vi "Motor-Maker-Triangle 2 RD.vi"() -> ()   [LabVIEW 2021]
panel:
  out "Motor Y\nLigado ida 2":bool=TRUE
  in  "stop Y descida":bool
  out "Posit Y descida":sgl
  out "Num Y descida":i32
  in  "Y descida":dbl
  out "Motor X\nLigado ida 3":bool=TRUE
  in  "stop X volta":bool
  out "Position X volta":sgl
  out "Nu X volta":i32
  in  "X volta":dbl
  out "Motor X\nLigado ida 2":bool=TRUE
  in  "stop X 2":bool
  out "pfPosition X ida 2":sgl
  out "Numeric X ida 2":i32
  in  "X ida 2":dbl
  out "Motor Y\nLigado ida":bool=TRUE
  in  "stop Y":bool
  out "Posit Y subida":sgl
  out "Num Y Subida":i32
  in  "Ysubida":dbl
  out "Motor X\nLigado ida":bool=TRUE
  in  "stop X":bool
  out "pfPosition X ida":sgl
  out "Numeric X ida":i32
  in  "X ida":dbl
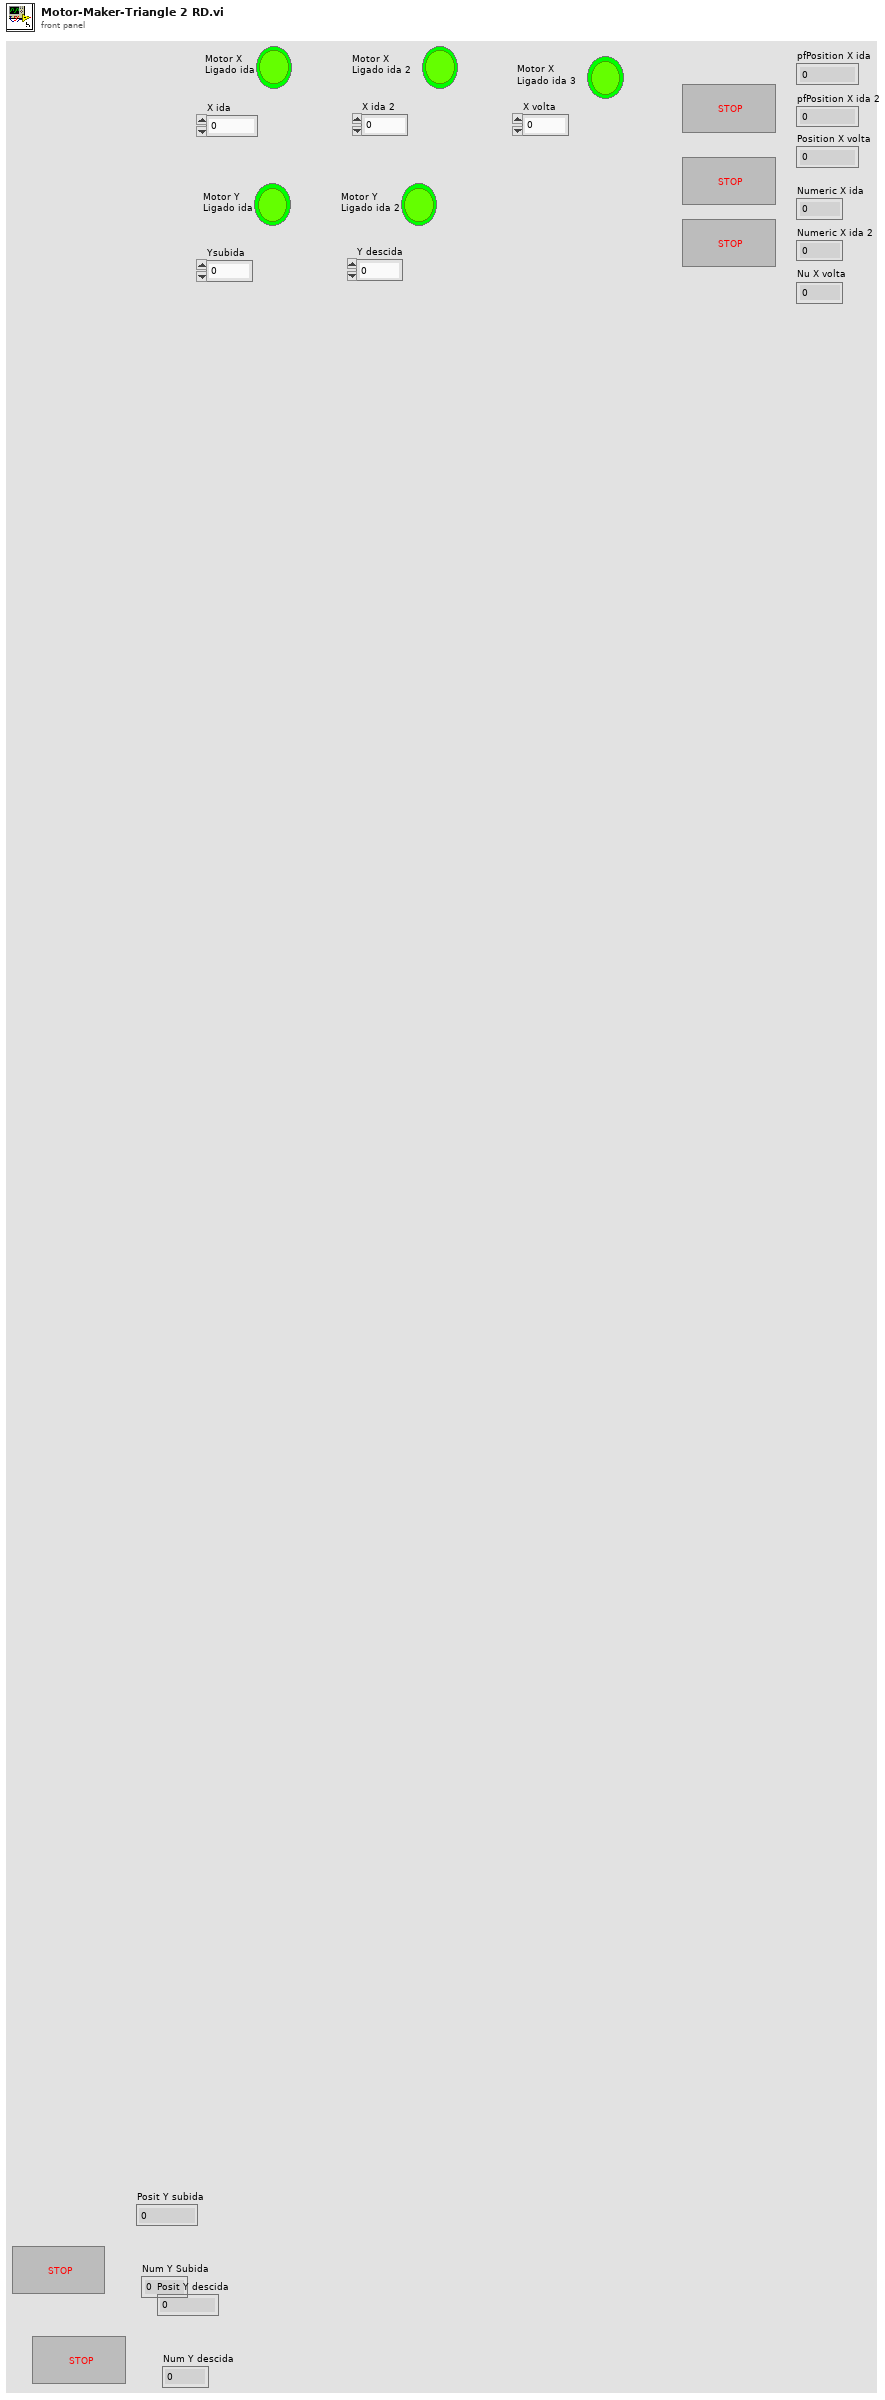
[diagram p1: front panel]
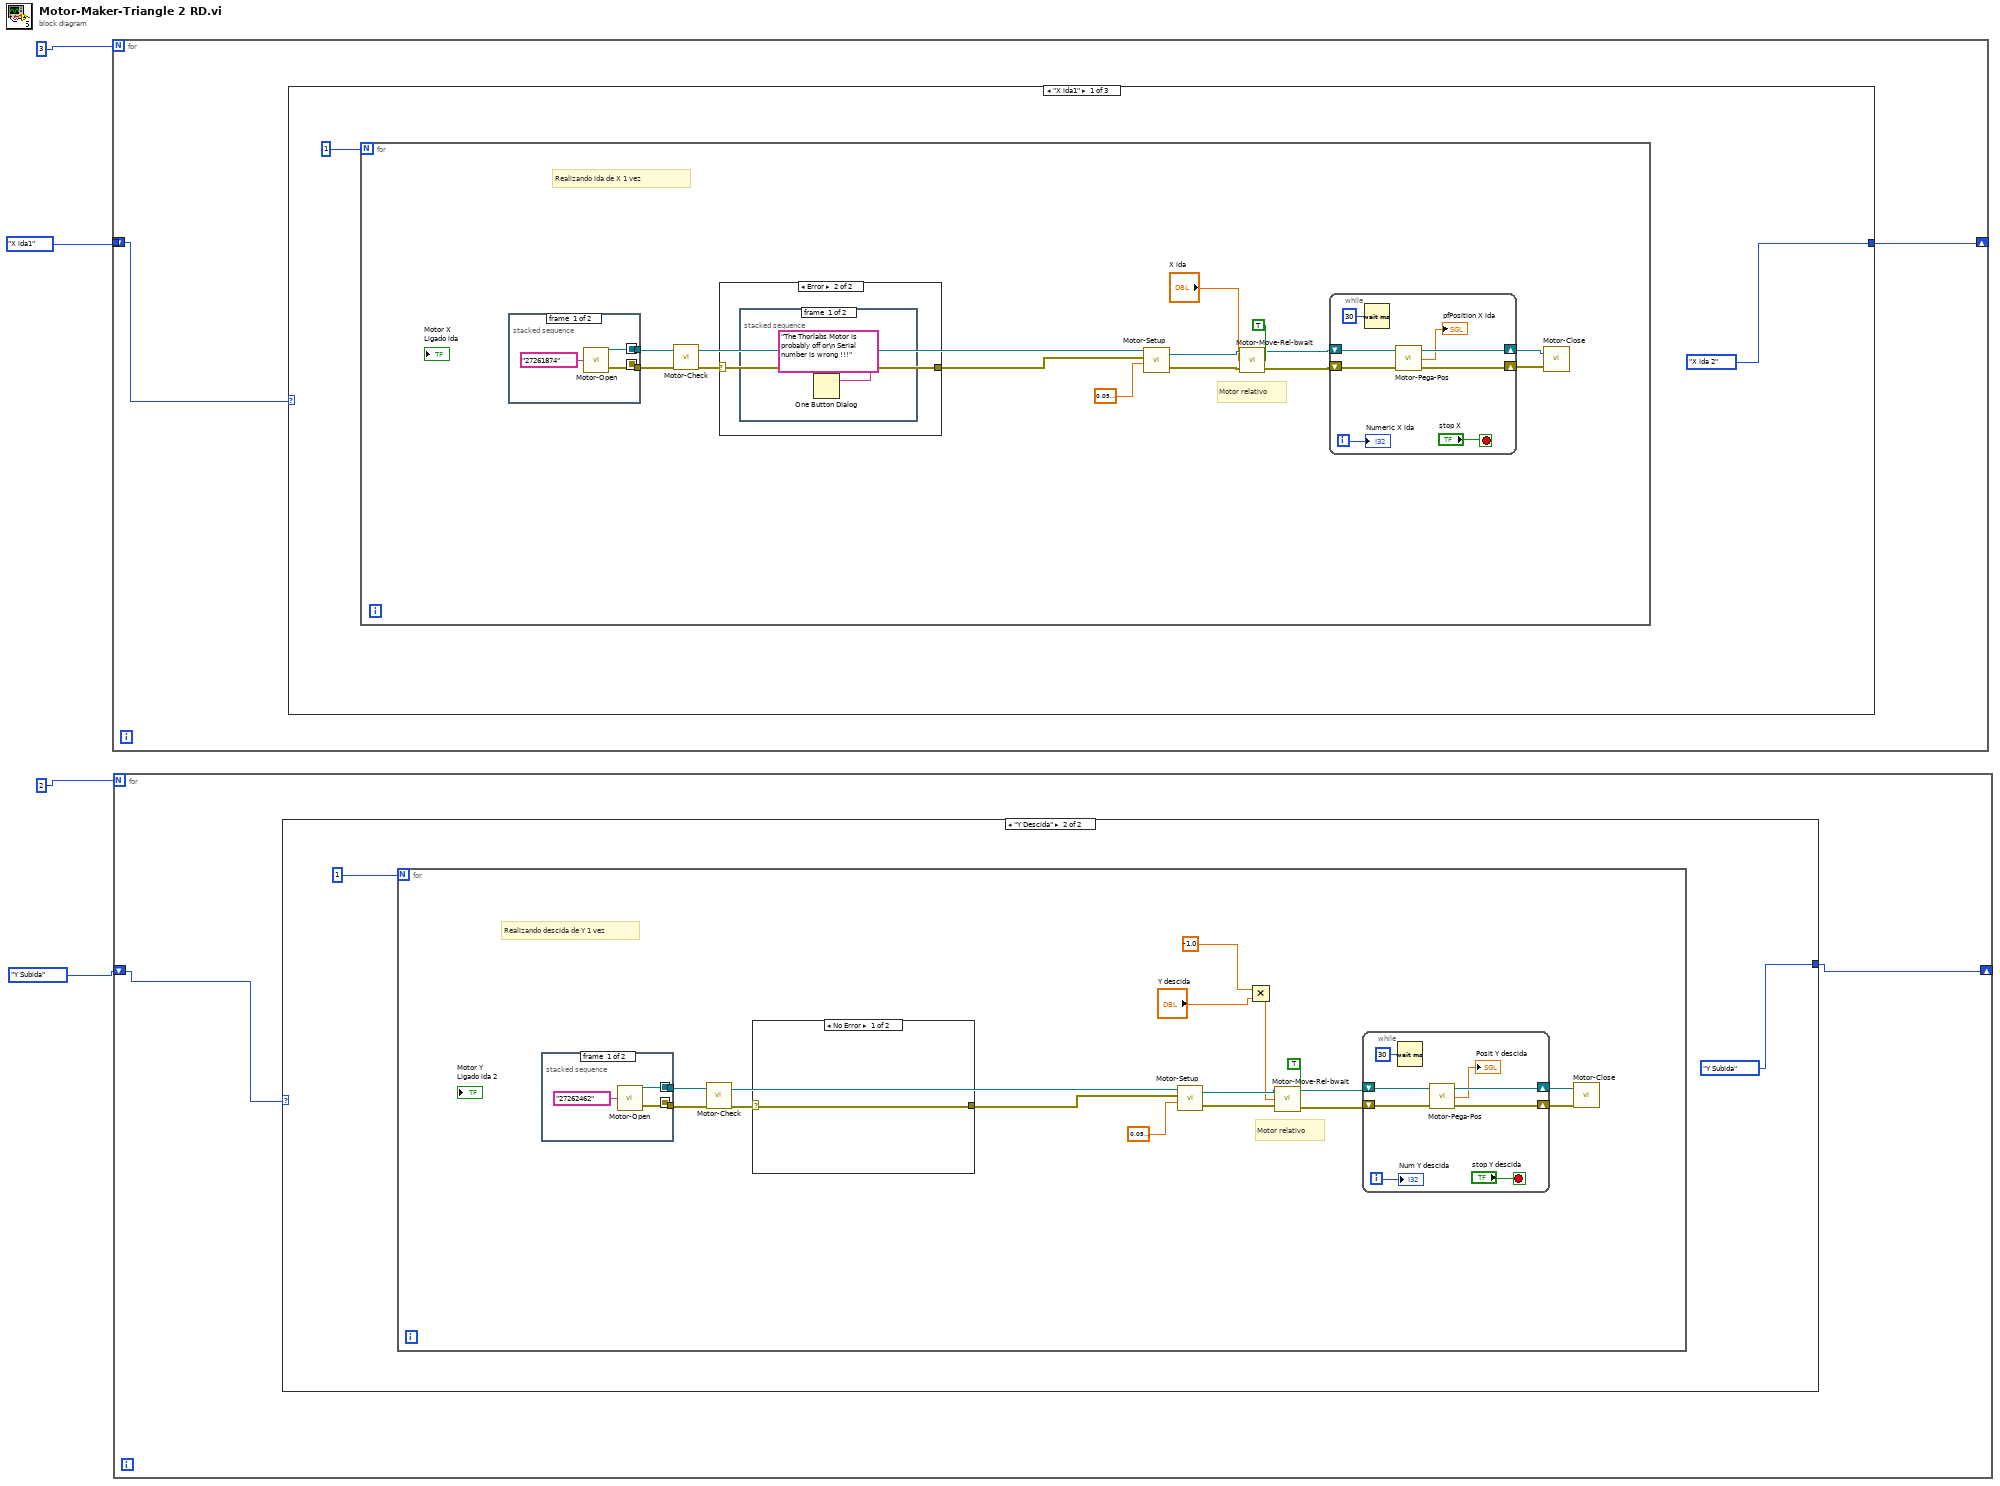
[diagram p0: block diagram]
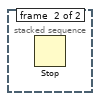
[diagram p3: hidden frame]
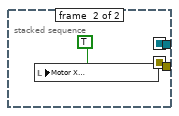
[diagram p4: hidden frame]
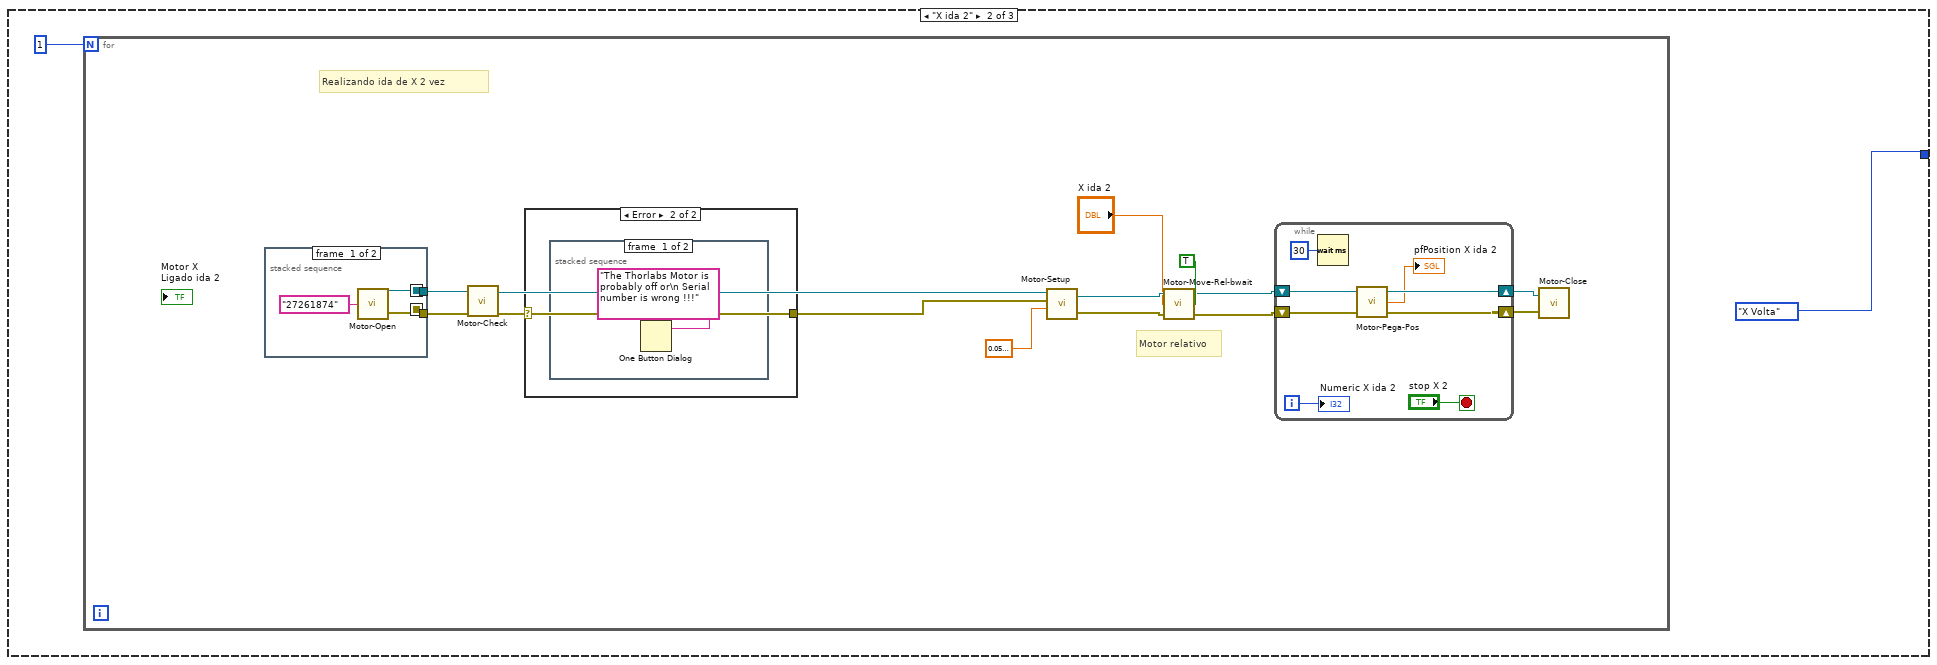
[diagram p5: hidden frame]
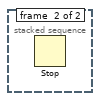
[diagram p7: hidden frame]
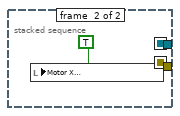
[diagram p8: hidden frame]
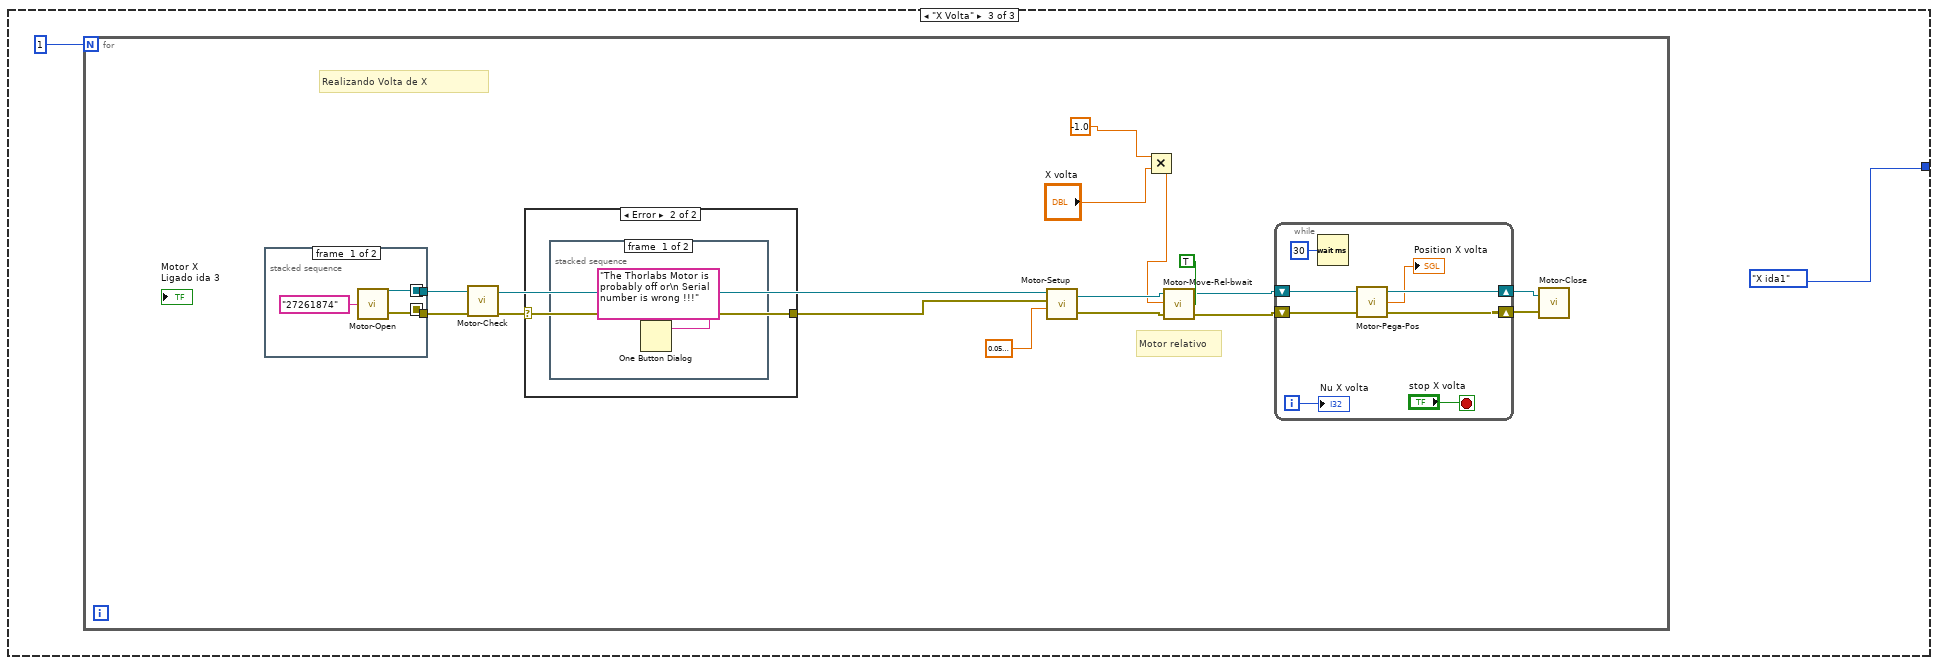
[diagram p9: hidden frame]
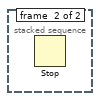
[diagram p11: hidden frame]
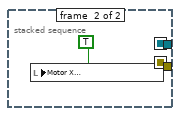
[diagram p12: hidden frame]
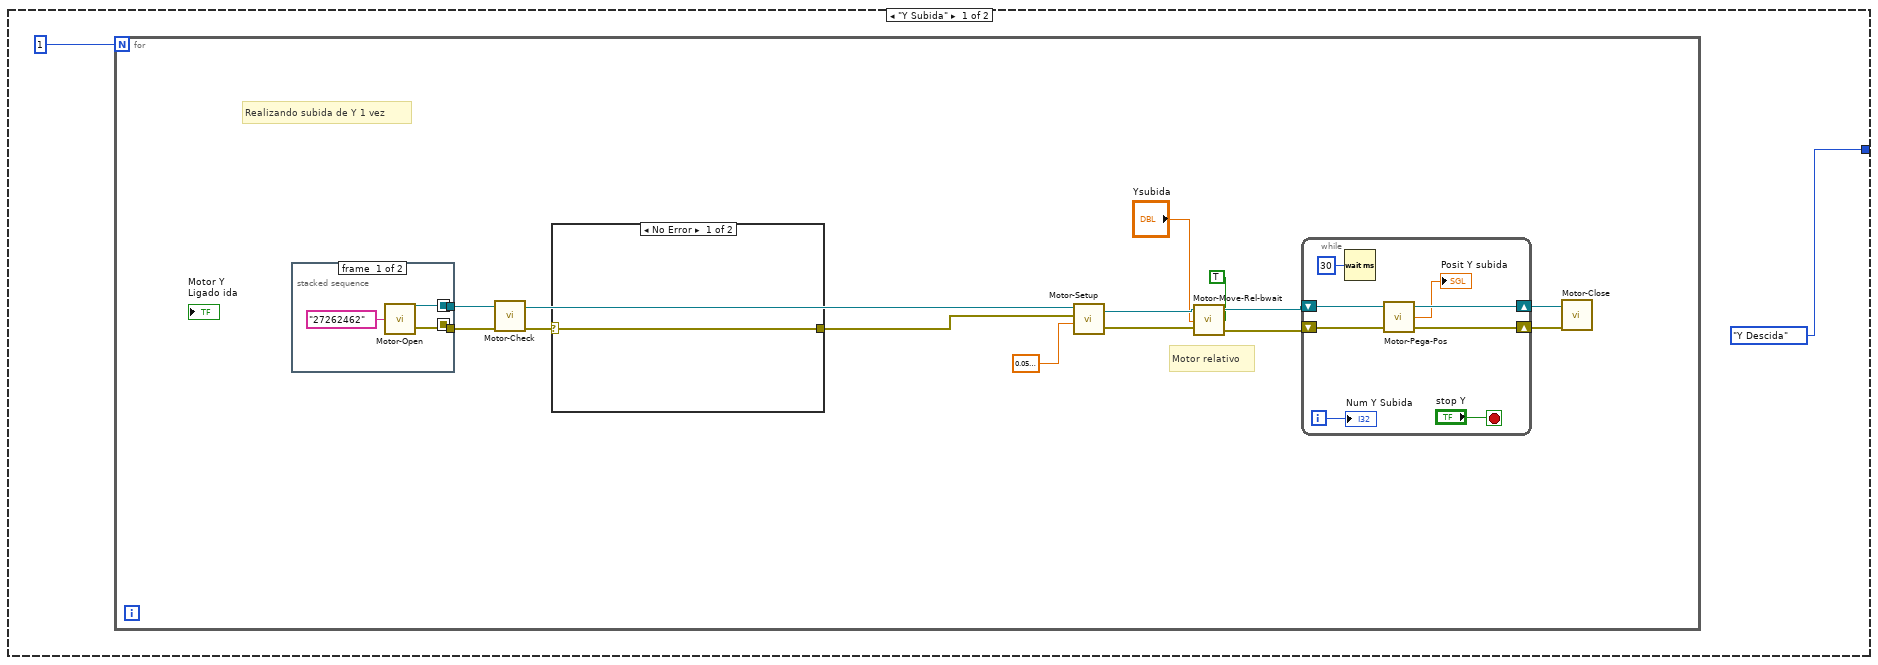
[diagram p13: hidden frame]
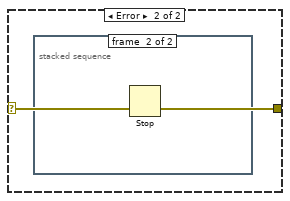
[diagram p14: hidden frame]
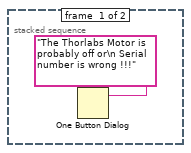
[diagram p15: hidden frame]
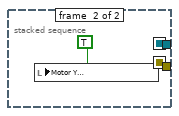
[diagram p16: hidden frame]
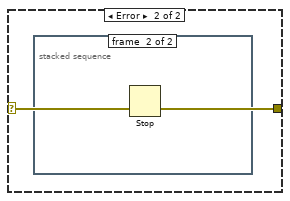
[diagram p17: hidden frame]
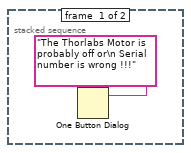
[diagram p18: hidden frame]
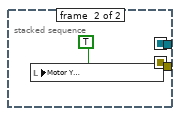
[diagram p19: hidden frame]
diagram:
  n1 = for {
    N: 3 -> [_]
    shift-right: [w6] -> _
    shift-left: _ -> [_]
    tunnel: enum16{"X ida1", "X Volta", "X ida 2"}."X ida1" -> [w5]
    n2 = case shown="\"X ida1\"" w5 {
      tunnel: [enum16{"X ida1", "X Volta", "X ida 2"}."X ida 2" enum16{"X ida1", "X Volta", "X ida 2"}."X Volta" enum16{"X ida1", "X Volta", "X ida 2"}."X ida1"] -> w6
      frame "X ida1" {
        n3 = for {
          N: 1 -> [_]
          # "Realizando ida de X 1 vez"
          # "Motor relativo"
          n4 = stacked-sequence {
            seq-local: [w36 _] -> [_ w39]
            seq-local: [w35 _] -> [_ w38]
            tunnel: [_ w39] -> w22
            tunnel: [_ w38] -> w21
            frame #0 {
              n5 = call "Motor-Open.vi"("S/N Motor"="27261874") -> ("MG17Motor 2"=w36:refnum<k7>, "error out"=w35:errorcluster)
            }
            frame #1 {
              n6 = local write "Motor X\nLigado ida"(TRUE ("Motor3\nLigado")) -> ()
            }
          }
          n7 = call "Motor-Check.vi"("error in (no error)"=w21, "Automation Refnum in"=w22) -> ("error out"=w20:errorcluster, "Automation Refnum out"=w19:refnum<k7>)  [unwired: 8 in]
          n8 = case shown="Error" w20 {
            selector: w20 -> [w23 w24]
            tunnel: [w23 w24] -> w18
            frame No Error {
            }
            frame Error {
              n9 = stacked-sequence {
                frame #0 {
                  n10 = One Button Dialog(message="The Thorlabs Motor is probably off or\n Serial number is wrong !!!") -> ()  [unwired: 1 in, 1 out]
                }
                frame #1 {
                  n11 = Stop() -> ()  [unwired: 1 in]
                }
              }
            }
          }
          n12 = call "Motor-Setup.vi"("Velocidade"=sgl 0.05, "error"=w18, "MG17Motor A"=w19) -> ("error out"=w12:errorcluster, "MG17Motor out"=w13:refnum<k7>)  [unwired: 1 in]
          n13 = call "Motor-Move-Rel-bwait.vi"("bWait"=TRUE, "error"=w12, "Posição"="X ida", "MG17Motor A"=w13) -> ("error out"=w9:errorcluster, "MG17Motor out"=w10:refnum<k7>)
          n14 = while {
            shift-right: [w31] -> w15
            shift-left: w10 -> [w33]
            shift-right: [w30] -> w16
            shift-left: w9 -> [w32]
            i -> [w26]
            stop <- "stop X" stop-if-true
            n15 = Wait (ms)(milliseconds to wait=u32 30) -> ()  [unwired: 1 out]
            n16 = call "Motor-Pega-Pos.vi"("MG17Motor 2"=w33, "error out"=w32) -> ("MG17Motor 3"=w31:refnum<k7>, "pfPosition"=→"pfPosition X ida":sgl, "error out 2"=w30:errorcluster)
            "Numeric X ida" <- w26
          }
          n17 = call "Motor-Close.vi"("error out"=w16, "MG17Motor 3"=w15) -> ()  [unwired: 1 in]
        }
      }
      frame "X ida 2" {
        n18 = for {
          N: 1 -> [_]
          # "Realizando ida de X 2 vez"
          # "Motor relativo"
          n19 = stacked-sequence {
            seq-local: [w69 _] -> [_ w72]
            seq-local: [w68 _] -> [_ w71]
            tunnel: [_ w72] -> w55
            tunnel: [_ w71] -> w54
            frame #0 {
              n20 = call "Motor-Open.vi"("S/N Motor"="27261874") -> ("MG17Motor 2"=w69:refnum<k7>, "error out"=w68:errorcluster)
            }
            frame #1 {
              n21 = local write "Motor X\nLigado ida 2"(TRUE ("Motor3\nLigado")) -> ()
            }
          }
          n22 = call "Motor-Check.vi"("error in (no error)"=w54, "Automation Refnum in"=w55) -> ("error out"=w53:errorcluster, "Automation Refnum out"=w52:refnum<k7>)  [unwired: 8 in]
          n23 = case shown="Error" w53 {
            selector: w53 -> [w56 w57]
            tunnel: [w56 w57] -> w51
            frame No Error {
            }
            frame Error {
              n24 = stacked-sequence {
                frame #0 {
                  n25 = One Button Dialog(message="The Thorlabs Motor is probably off or\n Serial number is wrong !!!") -> ()  [unwired: 1 in, 1 out]
                }
                frame #1 {
                  n26 = Stop() -> ()  [unwired: 1 in]
                }
              }
            }
          }
          n27 = call "Motor-Setup.vi"("Velocidade"=sgl 0.05, "error"=w51, "MG17Motor A"=w52) -> ("error out"=w45:errorcluster, "MG17Motor out"=w46:refnum<k7>)  [unwired: 1 in]
          n28 = call "Motor-Move-Rel-bwait.vi"("bWait"=TRUE, "error"=w45, "Posição"="X ida 2", "MG17Motor A"=w46) -> ("error out"=w42:errorcluster, "MG17Motor out"=w43:refnum<k7>)
          n29 = while {
            shift-right: [w64] -> w48
            shift-left: w43 -> [w66]
            shift-right: [w63] -> w49
            shift-left: w42 -> [w65]
            i -> [w59]
            stop <- "stop X 2" stop-if-true
            n30 = Wait (ms)(milliseconds to wait=u32 30) -> ()  [unwired: 1 out]
            n31 = call "Motor-Pega-Pos.vi"("MG17Motor 2"=w66, "error out"=w65) -> ("MG17Motor 3"=w64:refnum<k7>, "pfPosition"=→"pfPosition X ida 2":sgl, "error out 2"=w63:errorcluster)
            "Numeric X ida 2" <- w59
          }
          n32 = call "Motor-Close.vi"("error out"=w49, "MG17Motor 3"=w48) -> ()  [unwired: 1 in]
        }
      }
      frame "X Volta" {
        n33 = for {
          N: 1 -> [_]
          # "Realizando Volta de X"
          # "Motor relativo"
          n34 = stacked-sequence {
            seq-local: [w104 _] -> [_ w107]
            seq-local: [w103 _] -> [_ w106]
            tunnel: [_ w107] -> w90
            tunnel: [_ w106] -> w89
            frame #0 {
              n35 = call "Motor-Open.vi"("S/N Motor"="27261874") -> ("MG17Motor 2"=w104:refnum<k7>, "error out"=w103:errorcluster)
            }
            frame #1 {
              n36 = local write "Motor X\nLigado ida 3"(TRUE ("Motor3\nLigado")) -> ()
            }
          }
          n37 = call "Motor-Check.vi"("error in (no error)"=w89, "Automation Refnum in"=w90) -> ("error out"=w88:errorcluster, "Automation Refnum out"=w87:refnum<k7>)  [unwired: 8 in]
          n38 = case shown="Error" w88 {
            selector: w88 -> [w91 w92]
            tunnel: [w91 w92] -> w86
            frame No Error {
            }
            frame Error {
              n39 = stacked-sequence {
                frame #0 {
                  n40 = One Button Dialog(message="The Thorlabs Motor is probably off or\n Serial number is wrong !!!") -> ()  [unwired: 1 in, 1 out]
                }
                frame #1 {
                  n41 = Stop() -> ()  [unwired: 1 in]
                }
              }
            }
          }
          n42 = call "Motor-Setup.vi"("Velocidade"=sgl 0.05, "error"=w86, "MG17Motor A"=w87) -> ("error out"=w80:errorcluster, "MG17Motor out"=w81:refnum<k7>)  [unwired: 1 in]
          n43 = Multiply(x=-1.0, y="X volta") -> (x*y=w75:dbl)
          n44 = call "Motor-Move-Rel-bwait.vi"("bWait"=TRUE, "error"=w80, "Posição"=w75, "MG17Motor A"=w81) -> ("error out"=w78:errorcluster, "MG17Motor out"=w79:refnum<k7>)
          n45 = while {
            shift-right: [w99] -> w83
            shift-left: w79 -> [w101]
            shift-right: [w98] -> w84
            shift-left: w78 -> [w100]
            i -> [w94]
            stop <- "stop X volta" stop-if-true
            n46 = Wait (ms)(milliseconds to wait=u32 30) -> ()  [unwired: 1 out]
            n47 = call "Motor-Pega-Pos.vi"("MG17Motor 2"=w101, "error out"=w100) -> ("MG17Motor 3"=w99:refnum<k7>, "pfPosition"=→"Position X volta":sgl, "error out 2"=w98:errorcluster)
            "Nu X volta" <- w94
          }
          n48 = call "Motor-Close.vi"("error out"=w84, "MG17Motor 3"=w83) -> ()  [unwired: 1 in]
        }
      }
    }
  }
  n49 = for {
    N: 2 -> [_]
    shift-right: [w108] -> _
    shift-left: enum16{"Y Subida", "Y Descida"}."Y Subida" -> [w109]
    n50 = case shown="\"Y Descida\"" w109 {
      tunnel: [enum16{"Y Subida", "Y Descida"}."Y Descida" enum16{"Y Subida", "Y Descida"}."Y Subida"] -> w108
      frame "Y Subida" {
        n51 = for {
          N: 1 -> [_]
          # "Realizando subida de Y 1 vez"
          # "Motor relativo"
          n52 = stacked-sequence {
            seq-local: [w139 _] -> [_ w142]
            seq-local: [w138 _] -> [_ w141]
            tunnel: [_ w142] -> w123
            tunnel: [_ w141] -> w122
            frame #0 {
              n53 = call "Motor-Open.vi"("S/N Motor"="27262462") -> ("MG17Motor 2"=w139:refnum<k7>, "error out"=w138:errorcluster)
            }
            frame #1 {
              n54 = local write "Motor Y\nLigado ida"(TRUE ("Motor3\nLigado")) -> ()
            }
          }
          n55 = call "Motor-Check.vi"("error in (no error)"=w122, "Automation Refnum in"=w123) -> ("error out"=w121:errorcluster, "Automation Refnum out"=w120:refnum<k7>)  [unwired: 8 in]
          n56 = case shown="No Error" w121 {
            selector: w121 -> [w126 w127]
            tunnel: [w126 w127] -> w119
            frame No Error {
            }
            frame Error {
              n57 = stacked-sequence {
                frame #0 {
                  n58 = One Button Dialog(message="The Thorlabs Motor is probably off or\n Serial number is wrong !!!") -> ()  [unwired: 1 in, 1 out]
                }
                frame #1 {
                  n59 = Stop() -> ()  [unwired: 1 in]
                }
              }
            }
          }
          n60 = call "Motor-Setup.vi"("Velocidade"=sgl 0.05, "error"=w119, "MG17Motor A"=w120) -> ("error out"=w116:errorcluster, "MG17Motor out"=w117:refnum<k7>)  [unwired: 1 in]
          n61 = call "Motor-Move-Rel-bwait.vi"("bWait"=TRUE, "error"=w116, "Posição"="Ysubida", "MG17Motor A"=w117) -> ("error out"=w115:errorcluster, "MG17Motor out"=w113:refnum<k7>)
          n62 = while {
            shift-right: [w134] -> w125
            shift-left: w113 -> [w136]
            shift-right: [w133] -> w124
            shift-left: w115 -> [w135]
            i -> [w129]
            stop <- "stop Y" stop-if-true
            n63 = Wait (ms)(milliseconds to wait=u32 30) -> ()  [unwired: 1 out]
            n64 = call "Motor-Pega-Pos.vi"("MG17Motor 2"=w136, "error out"=w135) -> ("MG17Motor 3"=w134:refnum<k7>, "pfPosition"=→"Posit Y subida":sgl, "error out 2"=w133:errorcluster)
            "Num Y Subida" <- w129
          }
          n65 = call "Motor-Close.vi"("error out"=w124, "MG17Motor 3"=w125) -> ()  [unwired: 1 in]
        }
      }
      frame "Y Descida" {
        n66 = for {
          N: 1 -> [_]
          # "Realizando descida de Y 1 vez"
          # "Motor relativo"
          n67 = stacked-sequence {
            seq-local: [w174 _] -> [_ w177]
            seq-local: [w173 _] -> [_ w176]
            tunnel: [_ w177] -> w158
            tunnel: [_ w176] -> w157
            frame #0 {
              n68 = call "Motor-Open.vi"("S/N Motor"="27262462") -> ("MG17Motor 2"=w174:refnum<k7>, "error out"=w173:errorcluster)
            }
            frame #1 {
              n69 = local write "Motor Y\nLigado ida 2"(TRUE ("Motor3\nLigado")) -> ()
            }
          }
          n70 = call "Motor-Check.vi"("error in (no error)"=w157, "Automation Refnum in"=w158) -> ("error out"=w156:errorcluster, "Automation Refnum out"=w155:refnum<k7>)  [unwired: 8 in]
          n71 = case shown="No Error" w156 {
            selector: w156 -> [w161 w162]
            tunnel: [w161 w162] -> w154
            frame No Error {
            }
            frame Error {
              n72 = stacked-sequence {
                frame #0 {
                  n73 = One Button Dialog(message="The Thorlabs Motor is probably off or\n Serial number is wrong !!!") -> ()  [unwired: 1 in, 1 out]
                }
                frame #1 {
                  n74 = Stop() -> ()  [unwired: 1 in]
                }
              }
            }
          }
          n75 = call "Motor-Setup.vi"("Velocidade"=sgl 0.05, "error"=w154, "MG17Motor A"=w155) -> ("error out"=w151:errorcluster, "MG17Motor out"=w152:refnum<k7>)  [unwired: 1 in]
          n76 = Multiply(x=-1.0, y="Y descida") -> (x*y=w146:dbl)
          n77 = call "Motor-Move-Rel-bwait.vi"("bWait"=TRUE, "error"=w151, "Posição"=w146, "MG17Motor A"=w152) -> ("error out"=w150:errorcluster, "MG17Motor out"=w149:refnum<k7>)
          n78 = while {
            shift-right: [w169] -> w160
            shift-left: w149 -> [w171]
            shift-right: [w168] -> w159
            shift-left: w150 -> [w170]
            i -> [w164]
            stop <- "stop Y descida" stop-if-true
            n79 = Wait (ms)(milliseconds to wait=u32 30) -> ()  [unwired: 1 out]
            n80 = call "Motor-Pega-Pos.vi"("MG17Motor 2"=w171, "error out"=w170) -> ("MG17Motor 3"=w169:refnum<k7>, "pfPosition"=→"Posit Y descida":sgl, "error out 2"=w168:errorcluster)
            "Num Y descida" <- w164
          }
          n81 = call "Motor-Close.vi"("error out"=w159, "MG17Motor 3"=w160) -> ()  [unwired: 1 in]
        }
      }
    }
  }
